vi "introduction.vi"(1 "N":dbl) -> (0 "volume":dbl(slide) scale=0.0..1000.0)   [LabVIEW 2025]
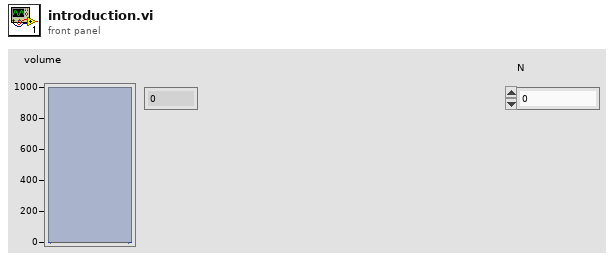
[diagram p1: front panel]
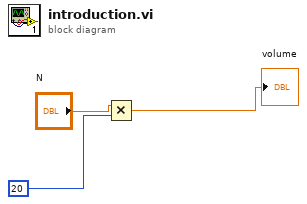
[diagram p0: block diagram]
diagram:
  n1 = Multiply(x="N", y=20) -> (x*y=→"volume":dbl)
